vi "Spex BurstControl.vi"() -> (3 "output 1":dbl)   [LabVIEW 2009]
uses:
  <vilib>/Instr/_visa.llb/VISA Configure Serial Port (Instr).vi
panel:
  in  "VISA resource name":refnum<visa-resource-name>="COM1"
  out "read buffer":string
  out "error out 4":errorcluster
  out "error out 3":errorcluster
  out "return count 3":u32
  out "Answer 2":string
  in  "Scan Type":bool=TRUE
  out "error buffer":string
  in  "String":string
  out "resulting string":string
  out "error out":errorcluster
  # "Normal"
  # "Trigger"
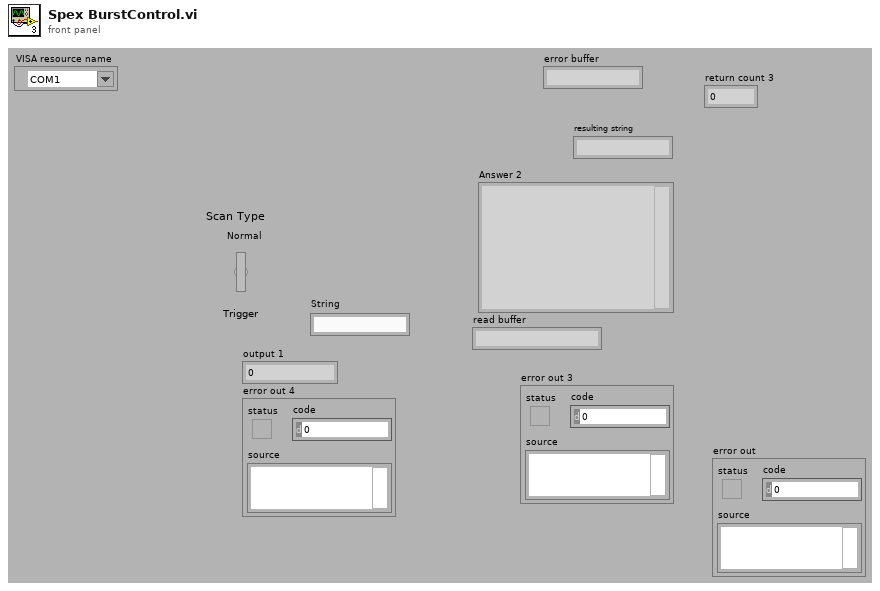
[diagram p1: front panel]
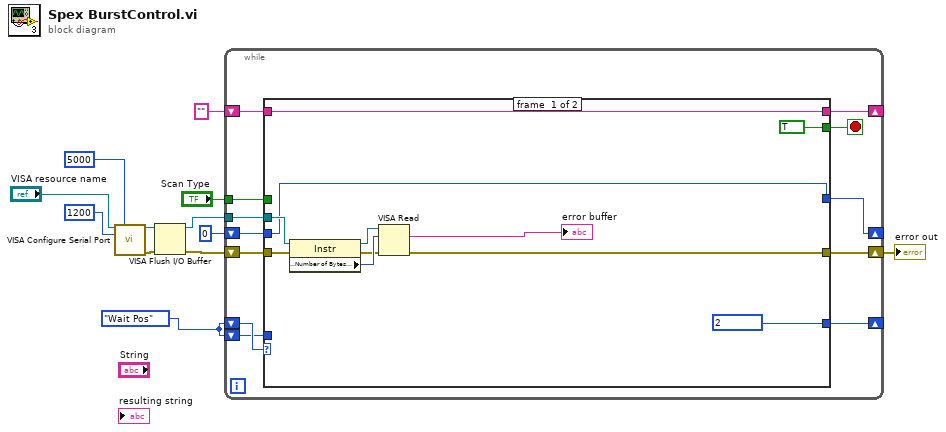
[diagram p0: block diagram]
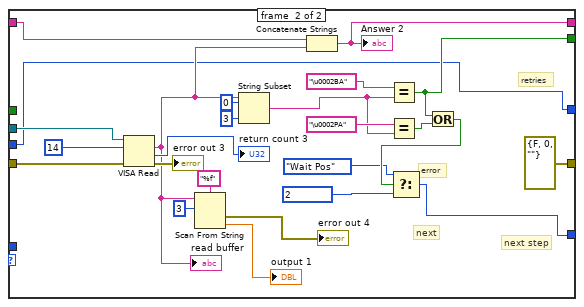
[diagram p2: hidden frame]
diagram:
  w1 = enum16{"Wait Pos", "Error"}."Wait Pos"
  n1 = call-poly "VISA Configure Serial Port"("VISA resource name"="VISA resource name", "timeout (10sec)"=u32 5000, "baud rate (9600)"=u32 1200) -> ("VISA resource name out"=w7:refnum<visa-resource-name>, "error out"=w8:errorcluster)  [unwired: 11 in]
  n2 = VISA Flush I/O Buffer(VISA resource name=w7, error in (no error)=w8) -> (VISA resource name out=w5:refnum<visa-resource-name>, error out=w6:errorcluster)  [unwired: 1 in]
  n3 = while {
    shift-right: [w16] -> _
    shift-left: w1 -> [w24]
    tunnel: w5 -> [w20]
    shift-right: [w22] -> w9
    shift-left: w6 -> [w23]
    shift-right: [w18] -> _
    shift-left: 0 -> [w19]
    shift-left: w1 -> [w17]
    tunnel: "Scan Type" -> [w15]
    shift-right: [w13] -> _
    shift-left: "" -> [w14]
    stop <- w21 stop-if-true
    n4 = case shown="\"Error\"" w24 {
      tunnel: w20 -> [w33 w56]
      tunnel: w23 -> [w34 w55]
      tunnel: [w29 errorcluster {"status"=FALSE, "code"=0, "source"=""} ("error out")] -> w22
      tunnel: [enum16{"Wait Pos", "Error"} 2 w40] -> w16
      tunnel: [TRUE w42] -> w21
      tunnel: w19 -> [w28 w39]
      tunnel: [w28 w39] -> w18
      tunnel: w17 -> [_ _]
      tunnel: w15 -> [_ _]
      tunnel: w14 -> [w27 w48]
      tunnel: [w27 w46] -> w13
      frame #0 {
        n5 = property class="Instr"(reference=w33, error in=w34) -> (reference out=w32:refnum<visa-resource-name>, error out=w30:errorcluster, "Serial Settings:Number of Bytes at Serial Port"=w31:u32)
        n6 = VISA Read(VISA resource name=w32, byte count=w31, error in (no error)=w30) -> (read buffer=→"error buffer":string, error out=w29:errorcluster)  [unwired: 2 out]
      }
      frame #1 {
        # "next"
        # "error"
        # "next step"
        # "retries"
        n7 = VISA Read(VISA resource name=w56, byte count=u32 14, error in (no error)=w55) -> (read buffer=w47:string, return count=→"return count 3":u32, error out=→"error out 3":errorcluster)  [unwired: 1 out]
        "read buffer" <- w47
        n8 = Scan From String(format string="%f", input string=w47, initial scan location=u32 3) -> (error out=→"error out 4":errorcluster, output 1=→"output 1":dbl)  [unwired: 2 in, 2 out]
        n9 = String Subset(string=w47, offset (0)=0, length (rest)=3 ("length (rest)")) -> (substring=w44:string)
        n10 = Concatenate Strings(w48, w47) -> (w46:string)
        "Answer 2" <- w46
        n11 = Equal?(x="\u0002BA", y=w44) -> (x = y?=w42:bool)
        n12 = Equal?(x="\u0002PA", y=w44) -> (x = y?=w43:bool)
        n13 = Or(x=w42, y=w43) -> (x .or. y?=w41:bool)
        n14 = Select(t=enum16{"Wait Pos", "Error"}."Wait Pos", s=w41, f=enum16{"Wait Pos", "Error"} 2) -> (s? t:f=w40:enum16{"Wait Pos", "Error"})
      }
    }
  }
  "error out" <- w9
